vi "Do.vi"(8 "error in (no error)":errorcluster, 10 "Actor in":refnum<class "Actor.lvclass">, 11 "Configure Arb Frequency [AF] Msg":refnum<class "Configure Arb Frequency [AF] Msg.lvclass">) -> (0 "error out":errorcluster, 2 "Actor out":refnum<class "Actor.lvclass">)   [LabVIEW 2015, in "CS++Fgen.lvlib" / "Configure Arb Frequency [AF] Msg.lvclass"]
doc: "This VI delivers the message to the actor by calling the appropriate method(s) on the actor."
uses:
  Configure Arb Frequency [AF] Msg.lvclass
  <vilib>/ActorFramework/Actor/Actor.lvclass
  CS++Fgen/CS++Fgen.lvclass
  CSPP_Core/Actors/CS++PVMonitor Messages/CS++PVUpdate Msg/CS++PVUpdate Msg.lvclass/CS++PVUpdate Msg.ctl
  CSPP_Core/Classes/CS++ProcessVariables/ProcessVariable/PV.lvclass/PV.ctl
  Configure Arb Frequency [AF] Msg.lvclass/Configure Arb Frequency [AF] Msg.ctl
  CSPP_Core/Classes/CS++ProcessVariables/ProcessVariable/PV.lvclass
  CSPP_Core/Actors/CS++PVMonitor Messages/CS++PVUpdate Msg/CS++PVUpdate Msg.lvclass
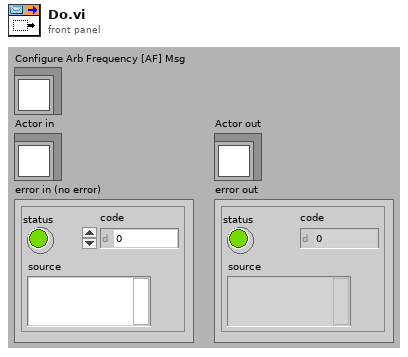
[diagram p1: front panel]
types:
  T1 = cluster{"channel name (\"CHANNEL1\")":string, "frequency (0.0 Hz)":dbl[unit]}
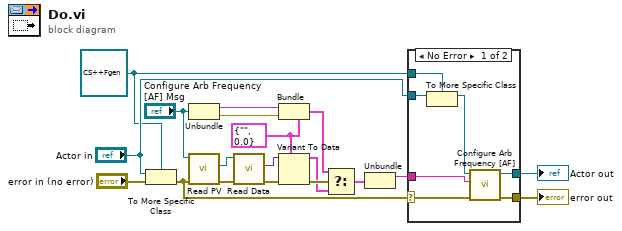
[diagram p0: block diagram]
diagram:
  w11 = T1 {"channel name (\"CHANNEL1\")"="", "frequency (0.0 Hz)"=0.0} ("Type")
  w15 = refnum<class "CS++Fgen.lvclass"> refnum ("Actor in")
  n1 = To More Specific Class(target class=w15, reference="Actor in", error in="error in (no error)") -> (error out=w4:errorcluster)  [unwired: 1 out]
  n2 = Unbundle ("Pre-Unbundler")("Configure Arb Frequency [AF] Msg") -> (w2:string, w1:dbl[unit])
  n3 = call "Read PV.vi"("error in (no error)"=w4, "CS++PVUpdate Msg in"="Configure Arb Frequency [AF] Msg") -> ("error out"=w14:errorcluster, "PV"=w10:refnum<class "PV.lvclass">)  [unwired: 7 in, 1 out]
  n4 = call "Read Data.vi"("error in (no error)"=w14, "PV in"=w10) -> ("error out"=w8:errorcluster, "Data"=w9:variant)  [unwired: 7 in, 1 out]
  n5 = Bundle ("Pre-Bundler")(cluster=w11, "channel name (\"CHANNEL1\")"=w2, "frequency (0.0 Hz)"=w1) -> (w12:T1)
  n6 = Variant To Data(error in=w8, type=w11, Variant=w9) -> (data=w6:T1, error out=w13:errorcluster)
  n7 = Select ("MainSelect")(t=w12, s=w13, f=w6) -> (s? t:f=w7:T1)
  n8 = Unbundle ("Main-Unbundler")(w7) -> ("channel name (\"CHANNEL1\")"=w3:string)  [unwired: 1 out]
  n9 = case shown="No Error" w4 {
    selector: w4 -> [w24 w28]
    tunnel: [w26 w28] -> w18
    tunnel: [w25 w27] -> w17
    tunnel: "Actor in" -> [w23 w27]
    tunnel: w15 -> [w22 _]
    tunnel: w3 -> [w20 _]
    frame No Error {
      n10 = To More Specific Class(target class=w22, reference=w23) -> (specific class reference=w21:refnum<class "CS++Fgen.lvclass">)  [unwired: 1 in, 1 out]
      n11 = call "Configure Arb Frequency [AF].vi"("error in (no error)"=w24, "channel name (\"CHANNEL1\")"=w20, "CS++Fgen in"=w21) -> ("error out"=w26:errorcluster, "CS++Fgen out"=w25:refnum<class "CS++Fgen.lvclass">)  [unwired: 7 in]
    }
    frame Error {
    }
  }
  "error out" <- w18
  "Actor out" <- w17
